vi "Generate Exit Event.vi"(8 "error in (no error)":errorcluster) -> (0 "error out":errorcluster)   [LabVIEW 2019, in "GaitDAQ UI.lvlib"]
uses:
  GaitDAQ UI.lvlib
panel:
  # "Input"
  # "Output"
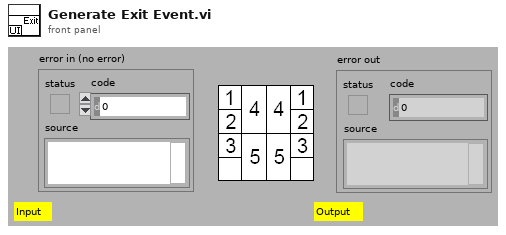
[diagram p1: front panel]
types:
  T1 = typedef "Event Message.lvlib/Event.ctl" = refnum<user-event>
  T2 = cluster{"Event Register Name":string, string, "variant":variant}
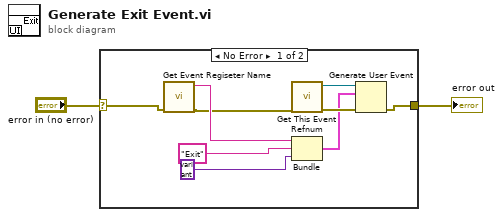
[diagram p0: block diagram]
diagram:
  n1 = case shown="No Error" "error in (no error)" {
    selector: "error in (no error)" -> [w3 w12]
    tunnel: [w9 w12] -> w1
    frame No Error {
      n2 = call "Get Event Regiseter Name.vi"("error in (no error)"=w3) -> ("error out"=w4:errorcluster, "Event Register Name"=w5:string)  [unwired: 9 in]
      n3 = call "Get This Event Refnum.vi"("error in (no error)"=w4) -> ("error out"=w10:errorcluster, "This Event Refnum Out"=w11:T1)  [unwired: 9 in]
      n4 = Bundle("Event Register Name"=w5, "Exit", "variant"=variant) -> (w6:T2)  [unwired: 1 in]
      n5 = Generate User Event(user event=w11, event data cluster=w6, error in=w10) -> (error out=w9:errorcluster)  [unwired: 1 in, 1 out]
    }
    frame Error {
    }
  }
  "error out" <- w1
